vi "json end.vi"(7 "input_str_product":string, 8 "input_str_CustomerPN":string, 9 "SN":string, 10 "FilePath":string, 11 "FileVer":string) -> (3 "midVar_Content":string)   [LabVIEW 2011]
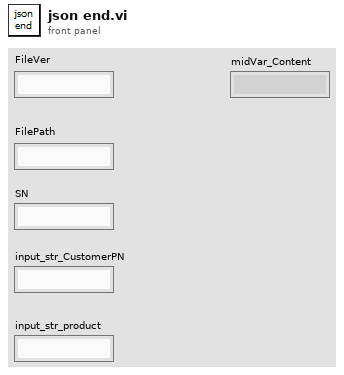
[diagram p1: front panel]
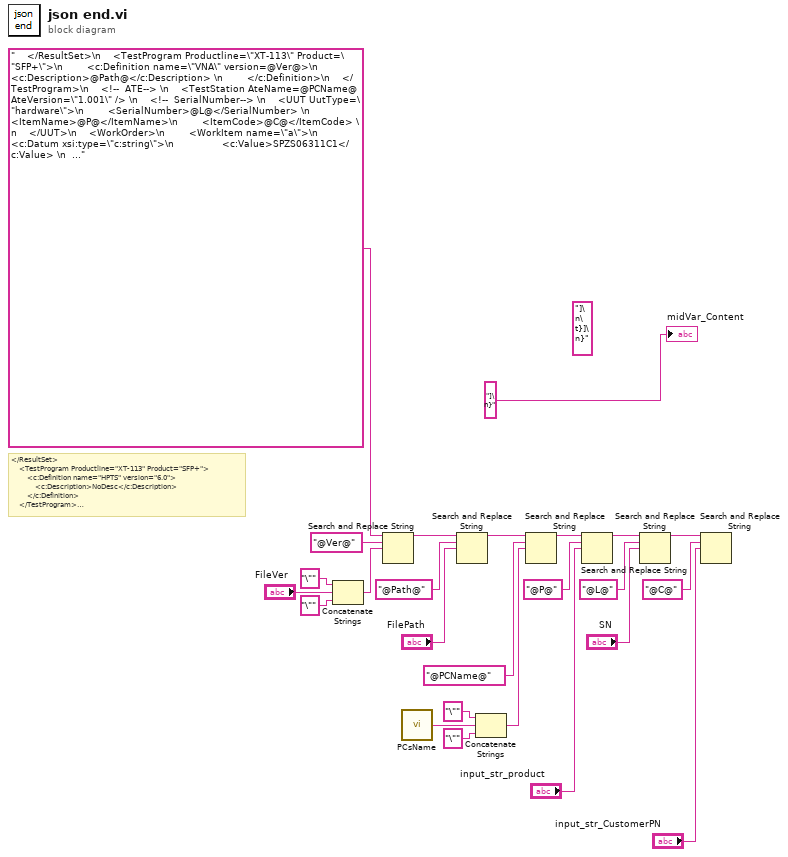
[diagram p0: block diagram]
diagram:
  (unwired) "]\n\t}]\n}"
  # "</ResultSet>\n    <TestProgram Productline=\"XT-113\" Product=\"SFP+\">\n        <c:Definition name=\"HPTS\" version=\"6.0\">\n            <c:Description>NoDesc</c:Description> \n        </c:Definition>\n    </TestProgram>\n    <!--  ATE--> \n    <TestStation AteName=\"TDR\" AteVersion=\"1.001\" /> \n    <!--  SerialNumber--> \n    <UUT UutType=\"hardware\">\n        <SerialNumber>@L@</SerialNumber> \n        <ItemName>SFP+</ItemName>\n        <ItemCode>@C@</ItemCode> \n    </UUT>\n    <WorkOrder>\n        <WorkItem name=\"a\">\n            <c:Datum xsi:type=\"c:string\">\n                <c:Value>SPZS06311C1</c:Value> \n            </c:Datum>\n        </WorkItem>\n    </WorkOrder>\n</TestResults"
  n1 = Concatenate Strings("\"" ("字符串"), "FileVer", "\"" ("字符串")) -> (w9:string)
  n2 = Search and Replace String(input string="    </ResultSet>\n    <TestProgram Productline=\"XT-113\" Product=\"SFP+\">\n        <c:Definition name=\"VNA\" version=@Ver@>\n            <c:Description>@Path@</c:Description> \n        </c:Definition>\n    </TestProgram>\n    <!--  ATE--> \n    <TestStation AteName=@PCName@ AteVersion=\"1.001\" /> \n    <!--  SerialNumber--> \n    <UUT UutType=\"hardware\">\n        <SerialNumber>@L@</SerialNumber> \n        <ItemName>@P@</ItemName>\n        <ItemCode>@C@</ItemCode> \n    </UUT>\n    <WorkOrder>\n        <WorkItem name=\"a\">\n            <c:Datum xsi:type=\"c:string\">\n                <c:Value>SPZS06311C1</c:Value> \n            </c:Datum>\n        </WorkItem>\n    </WorkOrder>\n</TestResults>", search string="@Ver@" ("搜索字符串"), replace string=w9) -> (result string=w18:string)  [unwired: 5 in, 3 out]
  n3 = call "PCsName.vi"() -> ("Computer Name"=w8:string)
  n4 = Search and Replace String(input string=w18, search string="@Path@" ("搜索字符串"), replace string="FilePath") -> (result string=w16:string)  [unwired: 5 in, 3 out]
  n5 = Concatenate Strings("\"" ("字符串"), w8, "\"" ("字符串")) -> (w5:string)
  n6 = Search and Replace String(input string=w16, search string="@PCName@" ("搜索字符串"), replace string=w5) -> (result string=w14:string)  [unwired: 5 in, 3 out]
  n7 = Search and Replace String(input string=w14, search string="@P@" ("搜索字符串"), replace string="input_str_product") -> (result string=w24:string)  [unwired: 5 in, 3 out]
  n8 = Search and Replace String(input string=w24, search string="@L@" ("搜索字符串"), replace string="SN") -> (result string=w22:string)  [unwired: 5 in, 3 out]
  n9 = Search and Replace String(input string=w22, search string="@C@" ("搜索字符串"), replace string="input_str_CustomerPN") -> ()  [unwired: 5 in, 4 out]
  "midVar_Content" <- "]\n}"
